vi "RM.setDeviceReservationDB.vi"(8 "error in":errorcluster, 10 "reservation DB in":variant, 11 "Item Ref in":T1 format="%.0x") -> (0 "error out":errorcluster, 1 "replaced":bool, 3 "Item Ref out":T1 format="%.0x")   [LabVIEW 2016, in "FPGA Resource Manager.lvlib"]
uses:
  FPGA Resource Manager.lvlib
  <vilib>/NI Veristand/Custom Device API/Custom Device Item Ref.ctl
  RM.Globals.vi
  <vilib>/NI Veristand/Custom Device API/Set Item Property (Variant).vi
  <vilib>/NI Veristand/Custom Device API/Custom Device API.lvlib
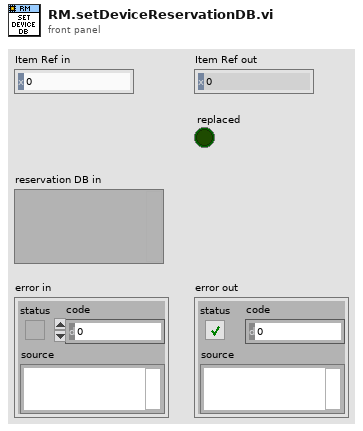
[diagram p1: front panel]
types:
  T1 = typedef "Custom Device API.lvlib/Custom Device Item Ref.ctl" = u64
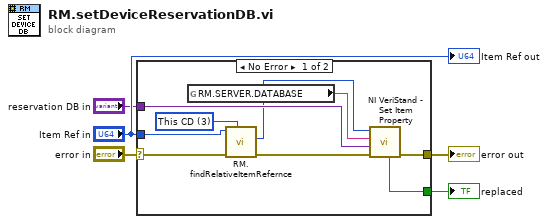
[diagram p0: block diagram]
diagram:
  n1 = case shown="No Error" "error in" {
    selector: "error in" -> [w8 w15]
    tunnel: "Item Ref in" -> [w10 _]
    tunnel: [w13 _] -> w5
    tunnel: [w14 w15] -> w3
    tunnel: "reservation DB in" -> [w12 _]
    frame No Error {
      w11 = u16 3 items=["Targets", "Controller", "Custom Devices", "This CD", "This CD/Group", "This CD/Group/SubGroup"] ("Relative Type")
      n2 = global read "RM.Globals.vi" "RM.SERVER.DATABASE"() -> (w6:string)
      n3 = call "RM.findRelativeItemRefernce.vi"("Relative Type"=w11, "error in (no error)"=w8, "Item Ref in"=w10) -> ("error out"=w7:errorcluster, "Relative Item Ref Out"=w9:T1)  [unwired: 4 in, 3 out]
      n4 = call-poly <vilib>:"NI VeriStand - Set Item Property.vi"("error in (no error)"=w7, "Value"=w12, "Property Name"=w6, "Item Ref in"=w9) -> ("error out"=w14:errorcluster, "Replaced"=w13:bool)  [unwired: 5 in, 1 out]
    }
    frame Error {
    }
  }
  "replaced" <- w5
  "error out" <- w3
  "Item Ref out" <- "Item Ref in"
